vi "Pockels Cal-Extract wavelength cal.vi"(8 "error in (no error)":errorcluster, 10 "Cal Wav listbox":refnum<vi>, 11 "All data loaded":string[][](array[string])) -> (0 "error IO":errorcluster, 2 "SINGLE CAL SET / Pockels Cal table (inc. headers & info)":string[][](array[string]))   [LabVIEW 2013]
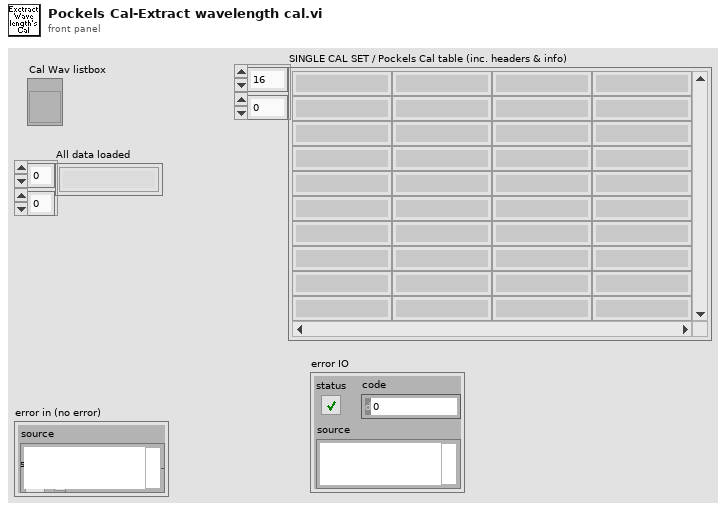
[diagram p1: front panel]
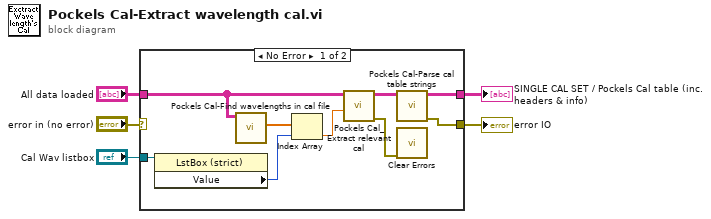
[diagram p0: block diagram]
diagram:
  n1 = case shown="No Error" "error in (no error)" {
    selector: "error in (no error)" -> [_ w15]
    tunnel: "All data loaded" -> [w13 _]
    tunnel: [w11 _] -> w3
    tunnel: "Cal Wav listbox" -> [w8 _]
    tunnel: [w6 w15] -> w2
    frame No Error {
      n2 = property on="Property Node" class="LstBox (strict)"(reference=w8) -> ("Value"=w9:i32)  [unwired: 1 in, 2 out]
      n3 = call "Pockels Cal-Find wavelengths in cal file.vi"("Loaded cal file"=w13) -> ("Pockels cal'd wavelengths"=w10:dbl[])  [unwired: 9 in, 1 out]
      n4 = Index Array(array=w10, index=w9) -> (element=w12:dbl)
      n5 = call "Pockels Cal_Extract relevant cal.vi"("Wavelength value"=w12, "Loaded table"=w13) -> ("error out"=w7:errorcluster, "Relevant cal only"=w14:string[][])  [unwired: 6 in, 2 out]
      n6 = call "Pockels Cal-Parse cal table strings.vi"("SINGLE CAL SET (inc. headers & info)"=w14) -> ("error out"=w6:errorcluster, "SINGLE CAL SET / Pockels Cal table (inc. headers & info)"=w11:string[][])  [unwired: 5 in, 4 out]
      n7 = call <vilib>:"Clear Errors.vi"("error in (no error)"=w7) -> ()  [unwired: 6 in, 1 out]
    }
    frame Error {
    }
  }
  "SINGLE CAL SET / Pockels Cal table (inc. headers & info)" <- w3
  "error IO" <- w2
